vi "printDirectory2.vi"(8 "Error In":errorcluster, 10 "nested level":u8, 11 "file":refnum<class "File.lvclass">) -> (0 "Error Out":errorcluster)   [LabVIEW 2014, in "LabVIEW Universal Transcriptor SD Card Library.lvlib"]
uses:
  LabVIEW Universal Transcriptor SD Card Library.lvlib
  File.lvclass
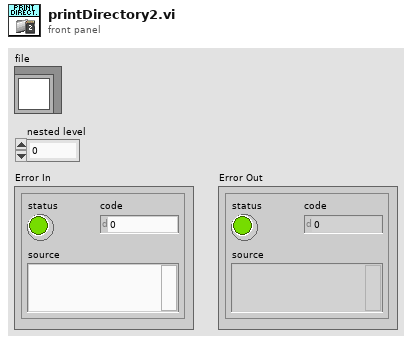
[diagram p1: front panel]
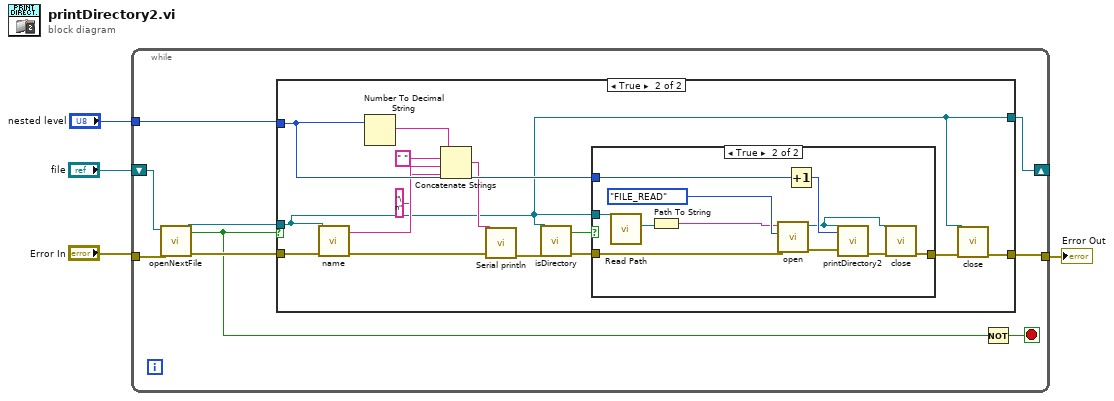
[diagram p0: block diagram]
diagram:
  n1 = while {
    tunnel: "nested level" -> [w10]
    tunnel: "Error In" -> [w7]
    tunnel: [w11] -> w3
    shift-right: [w6] -> _
    shift-left: "file" -> [w5]
    stop <- w9 stop-if-true
    n2 = call "openNextFile.vi"("error in (no error)"=w7, "File in"=w5) -> ("error out"=w12:errorcluster, "success?"=w8:bool, "File out"=w13:refnum<class "File.lvclass">)  [unwired: 7 in]
    n3 = case shown="True" w8 {
      tunnel: w13 -> [w14 w16]
      tunnel: w12 -> [w15 w29]
      tunnel: [w15 w19] -> w11
      tunnel: w10 -> [_ w24]
      tunnel: [w14 w16] -> w6
      frame False {
      }
      frame True {
        n4 = call-dynamic "name.vi"("error in (no error)"=w29, "File in"=w16) -> ("error out"=w28:errorcluster, "file name"=w18:string)  [unwired: 8 in]
        n5 = Number To Decimal String(number=w24) -> (decimal integer string=w23:string)  [unwired: 1 in]
        n6 = Concatenate Strings(w23, " " ("string"), w18, "\n" ("string")) -> (w21:string)
        n7 = call <vilib>:"Serial println.vi"("Error In"=w28, "string in"=w21) -> ("Error Out"=w27:errorcluster)  [unwired: 9 in]
        n8 = call-dynamic "isDirectory.vi"("error in (no error)"=w27, "File in"=w16) -> ("error out"=w26:errorcluster, "is directory?"=w25:bool)  [unwired: 8 in]
        n9 = case shown="True" w25 {
          tunnel: w26 -> [w30 w40]
          tunnel: [w30 w39] -> w20
          tunnel: w16 -> [_ w33]
          tunnel: w24 -> [_ w41]
          frame False {
          }
          frame True {
            n10 = call-dynamic "Read Path.vi"("File in"=w33) -> ("Path"=w32:path)  [unwired: 8 in, 2 out]
            n11 = Path To String(path=w32) -> (string=w31:string)
            n12 = call "open.vi"("Error In"=w40, "mode"=enum16{"FILE_READ", "FILE_WRITE"}."FILE_READ", "filepath"=w31) -> ("Error Out"=w36:errorcluster, "File out"=w34:refnum<class "File.lvclass">)  [unwired: 6 in, 1 out]
            n13 = Increment(x=w41) -> (x+1=w38:u8)
            n14 = call "printDirectory2.vi"("Error In"=w36, "nested level"=w38, "file"=w34) -> ("Error Out"=w35:errorcluster)  [unwired: 8 in]
            n15 = call-dynamic "close.vi"("error in (no error)"=w35, "File in"=w34) -> ("error out"=w39:errorcluster)  [unwired: 9 in]
          }
        }
        n16 = call-dynamic "close.vi"("error in (no error)"=w20, "File in"=w16) -> ("error out"=w19:errorcluster)  [unwired: 9 in]
      }
    }
    n17 = Not(x=w8) -> (.not. x?=w9:bool)
  }
  "Error Out" <- w3
